vi "Get Routing Channel State Configurations.vi"(8 "error in (no error)":errorcluster, 11 "Channel Ref in":T4 format="%.0x") -> (0 "error out":errorcluster, 2 "State Configurations":T1, 3 "Channel Ref out":T4=18446744073709551615 format="%.0x")   [LabVIEW 2017, in "Routing and Faulting Scripting.lvlib"]
uses:
  Routing and Faulting Scripting.lvlib
  <vilib>/NI Veristand/Custom Device API/Custom Device Item Ref.ctl
  Shared/Channel States.ctl
  Shared/Routing State.ctl
  Shared/Connection.ctl
  NationalInstruments.VeriStand.SystemDefinitionAPI
  Constants/Scripting Constants.vi
  Shared/Routing and Faulting Shared.lvlib
  <vilib>/NI VeriStand/Custom Device API/Custom Device API.lvlib
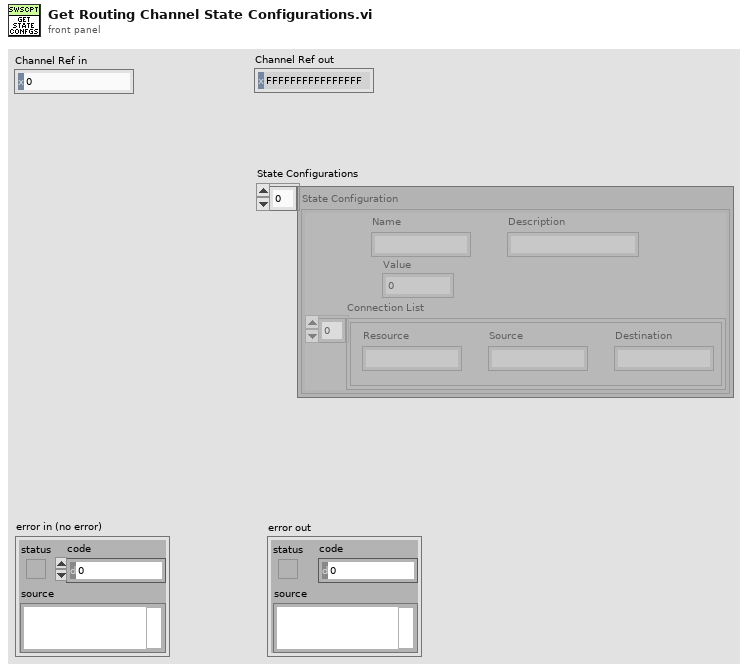
[diagram p1: front panel]
types:
  T1 = typedef "Routing and Faulting Shared.lvlib/Channel States.ctl" = T2[]
  T2 = typedef "Routing and Faulting Shared.lvlib/Routing State.ctl" = cluster{"Name":string, "Description":string, "Value":i32, "Connection List":T3[]}
  T3 = typedef "Routing and Faulting Shared.lvlib/Connection.ctl" = cluster{"Resource":string, "Source":string, "Destination":string}
  T4 = typedef "Custom Device API.lvlib/Custom Device Item Ref.ctl" = u64
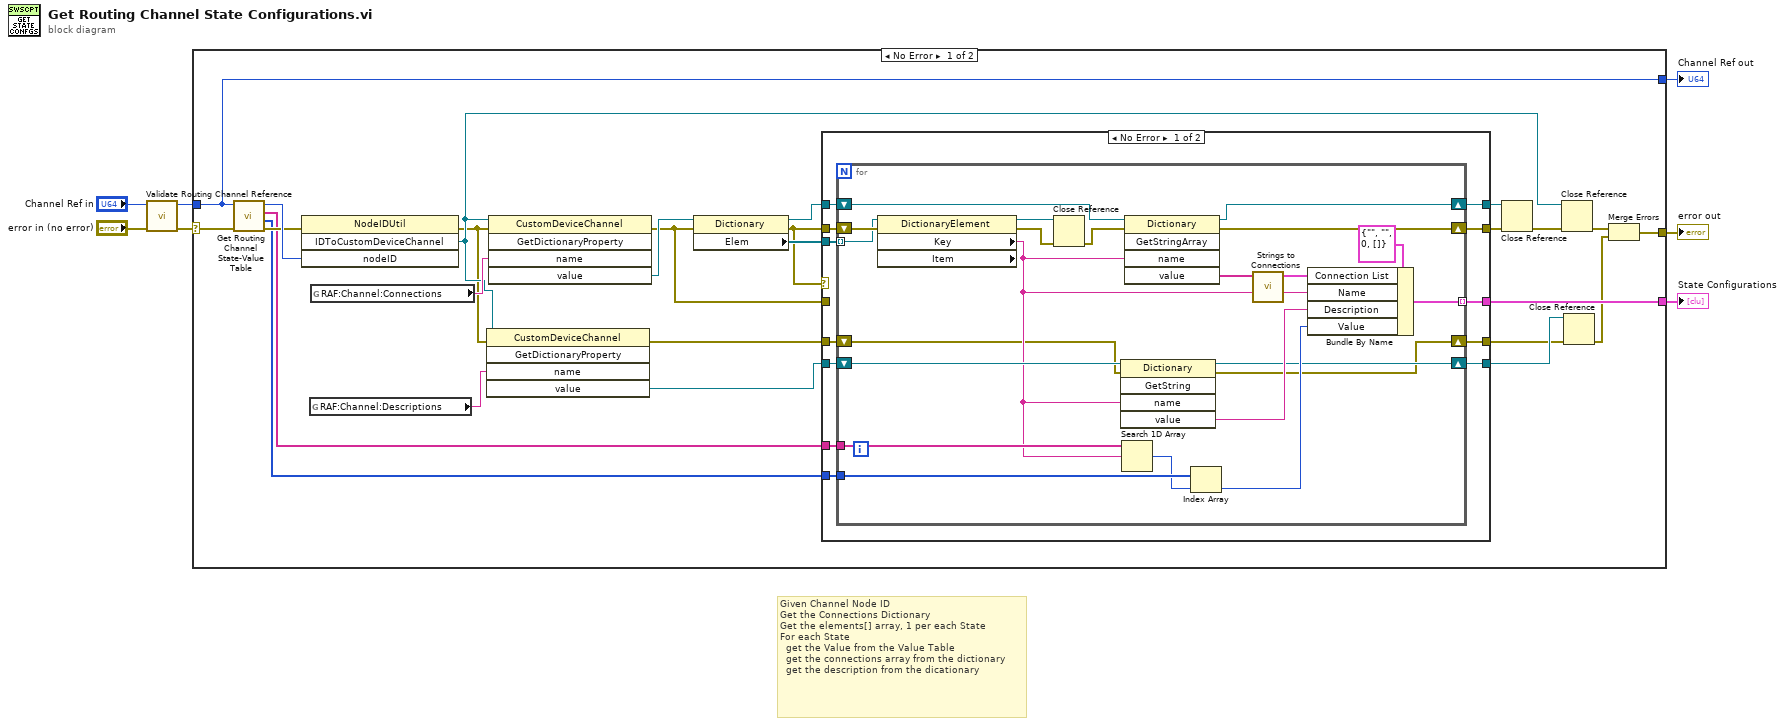
[diagram p0: block diagram]
diagram:
  # "Given Channel Node ID\nGet the Connections Dictionary\nGet the elements[] array, 1 per each State\nFor each State\n  get the Value from the Value Table\n  get the connections array from the dictionary\n  get the description from the dicationary"
  n1 = call "Validate Routing Channel Reference.vi"("error in (no error)"="error in (no error)", "Channel Ref in"="Channel Ref in") -> ("error out"=w3:errorcluster, "Channel Ref out"=w1:T4)  [unwired: 8 in]
  n2 = case shown="No Error" w3 {
    selector: w3 -> [w29 w73]
    tunnel: [w12 w73] -> w6
    tunnel: w1 -> [w8 w72]
    tunnel: [w8 w72] -> w5
    tunnel: [w31 _] -> w4
    frame No Error {
      n3 = call "Get Routing Channel State-Value Table.vi"("error in (no error)"=w29, "Channel Ref in"=w8) -> ("error out"=w28:errorcluster, "State Values"=w26:i32[], "State Names"=w27:string[], "Channel Ref out"=w30:T4)  [unwired: 6 in]
      n4 = invoke class="NodeIDUtil" method="IDToCustomDeviceChannel"(error in=w28, "nodeID"=w30) -> (error out=w18:errorcluster, "IDToCustomDeviceChannel"=w21:refnum<k24>)  [unwired: 2 in, 2 out]
      n5 = global read "Scripting Constants.vi" "RAF:Channel:Descriptions"() -> (w22:string)
      n6 = global read "Scripting Constants.vi" "RAF:Channel:Connections"() -> (w25:string)
      n7 = invoke class="CustomDeviceChannel" method="GetDictionaryProperty"(reference=w21, error in=w18, "name"=w22) -> (error out=w17:errorcluster, "value"=w20:refnum<k24>)  [unwired: 2 in, 3 out]
      n8 = invoke class="CustomDeviceChannel" method="GetDictionaryProperty"(reference=w21, error in=w18, "name"=w25) -> (error out=w9:errorcluster, "value"=w32:refnum<k24>)  [unwired: 2 in, 3 out]
      n9 = property class="Dictionary"(reference=w32, error in=w9) -> (reference out=w11:refnum<k24>, error out=w10:errorcluster, "Elem"=w23:refnum<k24>[])
      n10 = case shown="No Error" w10 {
        tunnel: [w45 w70] -> w33
        tunnel: w11 -> [w44 w71]
        tunnel: [w43 _] -> w31
        tunnel: w27 -> [w42 _]
        tunnel: w26 -> [w41 _]
        tunnel: w10 -> [w40 _]
        tunnel: [w39 w71] -> w24
        tunnel: w23 -> [w38 _]
        tunnel: w20 -> [w37 w68]
        tunnel: [w36 w68] -> w19
        tunnel: w17 -> [w35 w69]
        tunnel: [w34 w69] -> w16
        tunnel: w9 -> [_ w70]
        frame No Error {
          n11 = for {
            shift-right: [w52] -> w45
            shift-left: w40 -> [w64]
            shift-right: [w54] -> w39
            shift-left: w44 -> [w59]
            tunnel: w38 -> [w63] mode=indexing
            tunnel: [w67] -> w43 mode=indexing
            tunnel: w42 -> [w66]
            tunnel: w41 -> [w65]
            shift-right: [w50] -> w36
            shift-left: w37 -> [w53]
            shift-right: [w46] -> w34
            shift-left: w35 -> [w47]
            n12 = property class="DictionaryElement" props=["Key", "Item"](reference=w63, error in=w64) -> (reference out=w62:refnum<k24>, error out=w61:errorcluster, "Key"=w51:string)  [unwired: 1 out]
            n13 = Close Reference(reference=w62, error in (no error)=w61) -> (error out=w60:errorcluster)
            n14 = invoke class="Dictionary" method="GetString"(reference=w53, error in=w47, "name"=w51) -> (reference out=w50:refnum<k24>, error out=w46:errorcluster, "value"=w55:string)  [unwired: 2 in, 2 out]
            n15 = Search 1D Array(1D array=w66, element=w51) -> (index of element=w57:i32)  [unwired: 1 in]
            n16 = invoke class="Dictionary" method="GetStringArray"(reference=w59, error in=w60, "name"=w51) -> (reference out=w54:refnum<k24>, error out=w52:errorcluster, "value"=w49:string[])  [unwired: 2 in, 2 out]
            n17 = Index Array(array=w65, index=w57) -> (element=w56:i32)
            n18 = call "Strings to Connections.vi"("connection strings"=w49) -> ("connection list"=w48:T3[])  [unwired: 10 in]
            n19 = Bundle By Name(cluster=T2 {"Name"="", "Description"="", "Value"=0, "Connection List"=[]} ("Routing State"), "Connection List"=w48, "Name"=w51, "Description"=w55, "Value"=w56) -> (w67:T2)
          }
        }
        frame Error {
          # "Dictionary exists, but their are no elements at this point\nNo Connections have been added to the Dictionary."
        }
      }
      n20 = Close Reference(reference=w24, error in (no error)=w33) -> (error out=w15:errorcluster)
      n21 = Close Reference(reference=w21, error in (no error)=w15) -> (error out=w14:errorcluster)
      n22 = Close Reference(reference=w19, error in (no error)=w16) -> (error out=w13:errorcluster)
      n23 = Merge Errors(w14, w13) -> (w12:errorcluster)
    }
    frame Error {
    }
  }
  "Channel Ref out" <- w5
  "error out" <- w6
  "State Configurations" <- w4
